vi "Benchmark Logger.vi"() -> ()   [LabVIEW 2016]
uses:
  HSE-Logger/LogLevel.ctl
  HSE-Logger/Handler/FileHandler/FileHandler.lvclass/FileHandler.ctl
  <vilib>/Analysis/baseanly.llb/Mean (DBL).vi
  HSE-Logger/Formatter/JSONLFormatter/JSONLFormatter.lvclass
  C:/_work/hampel-soft/open-source/hse-logger/Source/HSE-Logger/Formatter/Formatter.lvclass
  HSE-Logger/Handler/FileHandler/FileHandler.lvclass
  C:/_work/hampel-soft/open-source/hse-logger/Source/HSE-Logger/Handler/Handler.lvclass
  HSE-Logger/hse-logger.lvlib
  <vilib>/Analysis/NI_AALBase.lvlib
  HSE-Logger/Formatter/Formatter.lvclass
panel:
  out "Logging performance (ms)":dbl[](graph)
  in  "Handler Type":enum16{"Standard", "JSONLines"}(ring)
  in  "Number of Handlers":u8=1 min=1
  out "Min (ms)":dbl
  out "Max (ms)":dbl
  out "Median (ms)":dbl format="%f"
  out "Mean (ms)":dbl format="%f"
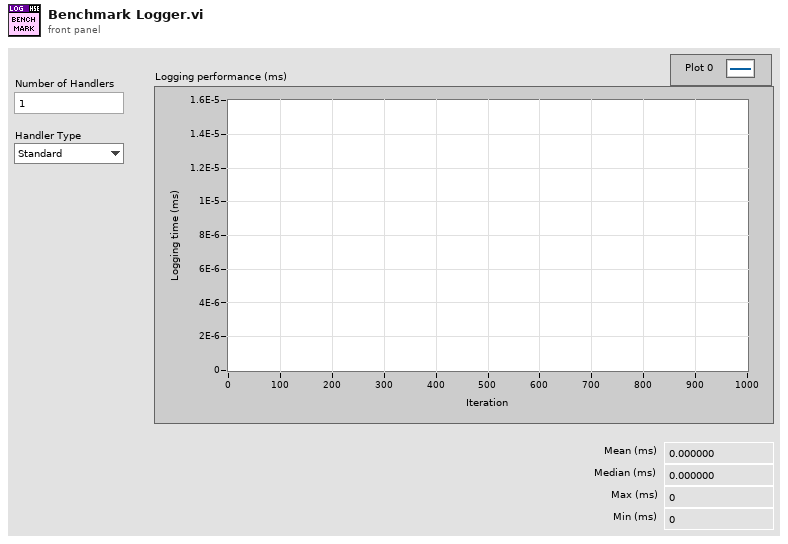
[diagram p1: front panel]
types:
  T1 = typedef "hse-logger.lvlib/LogLevel.ctl" = enum16{"DEBUG", "INFO", "WARNING", "ERROR", "CRITICAL"}
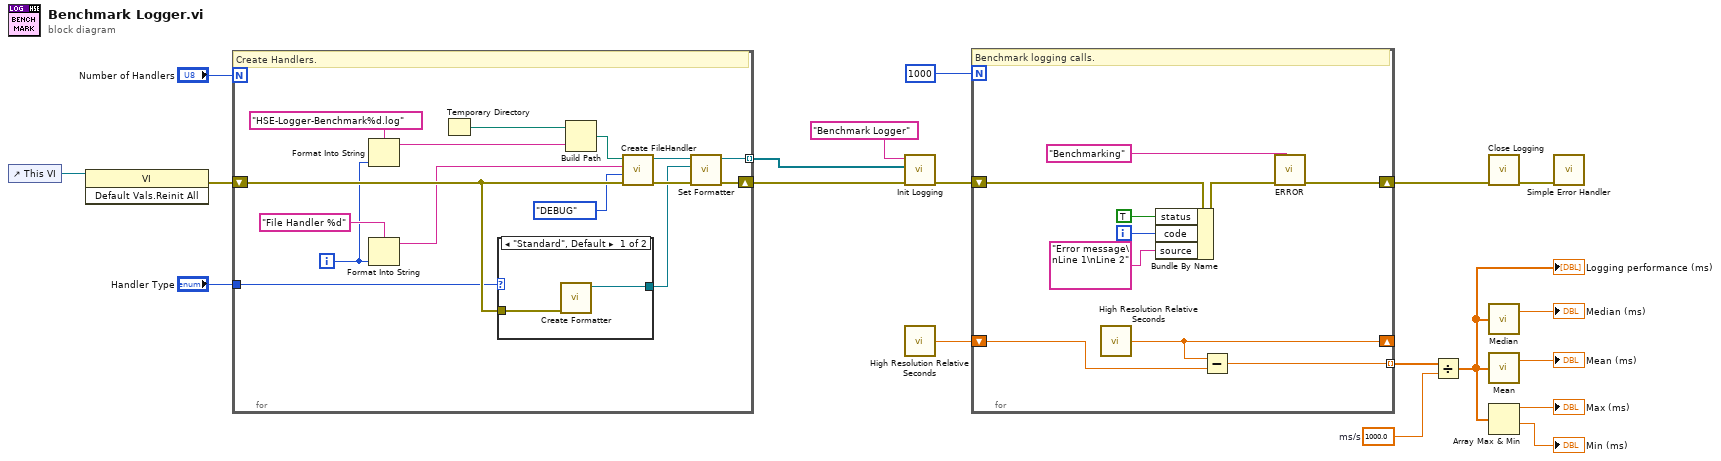
[diagram p0: block diagram]
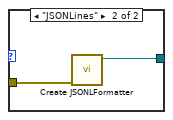
[diagram p2: hidden frame]
diagram:
  w5 = 1000.0  # ms/s
  n1 = control-ref of="This VI"() -> (w19:refnum<vi>)
  n2 = invoke class="VI" method="Default Vals.Reinit All"(reference=w19) -> (error out=w18:errorcluster)  [unwired: 2 in, 2 out]
  n3 = for {
    N: "Number of Handlers" -> [_]
    shift-right: [w28] -> w16
    shift-left: w18 -> [w34]
    tunnel: "Handler Type" -> [w26]
    tunnel: [w25] -> w2 mode=indexing
    i -> [w21]
    # "Create Handlers."
    n4 = Format Into String(format string="HSE-Logger-Benchmark%d.log" ("name or relative path"), w21) -> (resulting string=w20:string)  [unwired: 2 in, 1 out]
    n5 = Format Into String(format string="File Handler %d" ("Name"), w21) -> (resulting string=w23:string)  [unwired: 2 in, 1 out]
    n6 = Temporary Directory() -> (w32:path)
    n7 = case shown="\"Standard\", Default" w26 {
      tunnel: w34 -> [w35 w38]
      tunnel: [w36 w37] -> w27
      frame "Standard", Default {
        n8 = call "Create Formatter.vi"("error in"=w35) -> ("Formatter out"=w36:refnum<class "Formatter.lvclass">)  [unwired: 9 in, 1 out]
      }
      frame "JSONLines" {
        n9 = call "Create JSONLFormatter.vi"("error in"=w38) -> ("JSONLFormatter out"=w37:refnum<class "JSONLFormatter.lvclass">)  [unwired: 9 in, 1 out]
      }
    }
    n10 = Build Path(base path=w32, name or relative path=w20) -> (appended path=w31:path)
    n11 = call "Create FileHandler.vi"("error in"=w34, "Level"=LogLevel."DEBUG", "Name"=w23, "Filepath"=w31) -> ("error out"=w33:errorcluster, "FileHandler out"=w29:refnum<class "FileHandler.lvclass">)  [unwired: 6 in]
    n12 = call "Set Formatter.vi"("error in"=w33, "Formatter.lvclass"=w27, "FileHandler"=w29) -> ("error out"=w28:errorcluster, "FileHandler out"=w25:refnum<class "FileHandler.lvclass">)  [unwired: 7 in]
  }
  n13 = call "Init Logging.vi"("error in"=w16, "Handlers"=w2, "Name"="Benchmark Logger") -> ("error out"=w15:errorcluster)  [unwired: 8 in]
  n14 = call <vilib>:"High Resolution Relative Seconds.vi"() -> ("relative seconds"=w11:dbl)
  n15 = for {
    N: 1000 -> [_]
    shift-right: [w47] -> w14
    shift-left: w15 -> [w48]
    shift-right: [w40] -> _
    shift-left: w11 -> [w41]
    tunnel: [w39] -> w8 mode=indexing
    i -> [w44]
    # "Benchmark logging calls."
    n16 = call <vilib>:"High Resolution Relative Seconds.vi"() -> ("relative seconds"=w40:dbl)
    n17 = Bundle By Name(cluster=w48, "status"=TRUE, "code"=w44, "source"="Error message\nLine 1\nLine 2") -> (w46:errorcluster)
    n18 = Subtract(x=w40, y=w41) -> (x-y=w39:dbl)
    n19 = call "ERROR.vi"("Message"="Benchmarking", "error in"=w46) -> ("error out"=w47:errorcluster)  [unwired: 9 in]
  }
  n20 = Divide(x=w8, y=w5) -> (x/y=w1:dbl[])
  "Logging performance (ms)" <- w1
  n21 = call "Close Logging.vi"("error in"=w14) -> ("error out"=w13:errorcluster)  [unwired: 10 in]
  n22 = call <vilib>:"Median.vi"("X"=w1) -> ("median"=→"Median (ms)":dbl)  [unwired: 1 out]
  n23 = call-poly <vilib>:"Mean.vi"("X"=w1) -> ("mean"=→"Mean (ms)":dbl)  [unwired: 1 out]
  n24 = Array Max & Min(array=w1) -> (max value=→"Max (ms)":dbl, min value=→"Min (ms)":dbl)  [unwired: 2 out]
  n25 = call <vilib>:"Simple Error Handler.vi"("error in (no error)"=w13) -> ()  [unwired: 4 in, 5 out]
